vi "Reserve(Session).vi"(8 "error in (no error)":errorcluster, 10 "port":u32, 11 "board":u32) -> (0 "error out":errorcluster, 1 "found":bool, 2 "PortHandle":u32, 3 "BoardHandle":u32)   [LabVIEW 2020, in "AIM664LV.lvlib"]
uses:
  AIM664LV.lvlib
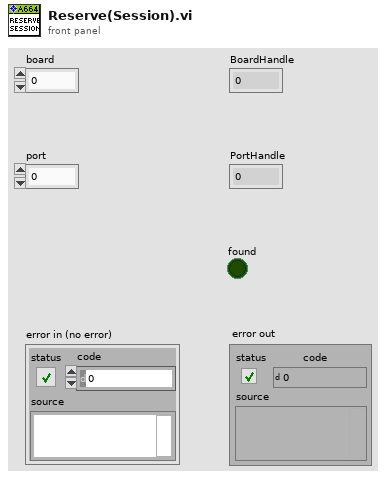
[diagram p1: front panel]
types:
  T1 = cluster{"ResourceID":u32, "ResourceType":u32, "ResourceInfo":string, "StructId":u32}
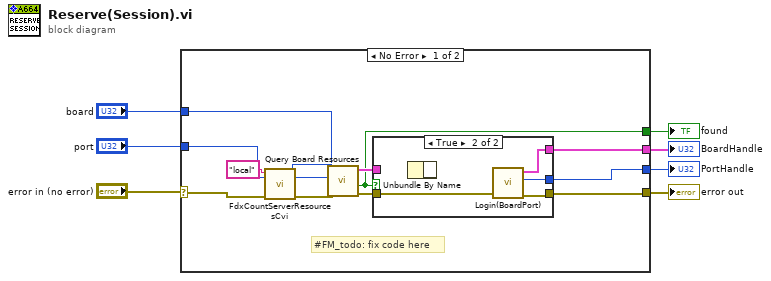
[diagram p0: block diagram]
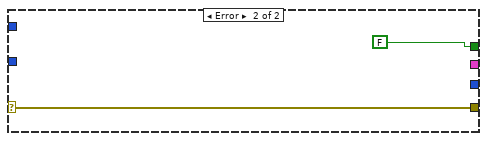
[diagram p3: hidden frame]
diagram:
  n1 = case shown="No Error" "error in (no error)" {
    selector: "error in (no error)" -> [w14 w25]
    tunnel: [w10 w25] -> w7
    tunnel: [w13 FALSE] -> w5
    tunnel: "board" -> [w12 _]
    tunnel: "port" -> [w11 _]
    tunnel: [w9 _] -> w2
    tunnel: [w8 _] -> w1
    frame No Error {
      # "#FM_todo: fix code here"
      n2 = call "FdxCountServerResourcesCvi.vi"("error in"=w14, "SrvName (local)"="local" ("SrvName(local)")) -> ("error out"=w17:errorcluster, "Number of Resources"=w18:u32)  [unwired: 8 in]
      n3 = call "Query Board Resources.vi"("error in (no error)"=w17, 9:w18, 10:w11, "board"=w12) -> ("error out"=w15:errorcluster, "found"=w13:bool, "board resource"=w16:T1)  [unwired: 5 in]
      n4 = case shown="True" w13 {
        tunnel: w16 -> [_ _]
        tunnel: w15 -> [w20 w24]
        tunnel: [w20 w23] -> w10
        tunnel: [_ w22] -> w8
        tunnel: [_ w21] -> w9
        frame False {
        }
        frame True {
          n5 = Unbundle By Name() -> ()  [unwired: 1 in, 1 out]
          n6 = call "Login(BoardPort).vi"("error in (no error)"=w24) -> ("error out"=w23:errorcluster, "Handle"=w22:u32, "resource out"=w21:T1)  [unwired: 8 in]
        }
      }
    }
    frame Error {
    }
  }
  "error out" <- w7
  "BoardHandle" <- w2
  "PortHandle" <- w1
  "found" <- w5
